vi "detect_spike_A_B_clean.vi"(6 "IO Module\\AI 1 Data N-3":i16, 9 "IO Module\\AI 1 Data N-2":i16, 10 "IO Module\\AI 1 Data N-1":i16, 11 "IO Module\\AI 1 Data N":i16) -> (3 "Numeric":i32, 5 "Read Ready A":bool, 7 "Read Ready B":bool)   [LabVIEW 2020]
panel:
  out "count_out":i16
  out "Read B 2":bool
  out "Read A 2":bool
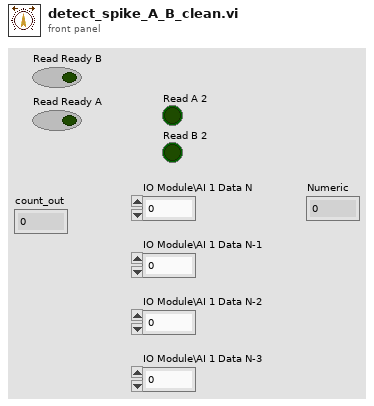
[diagram p1: front panel]
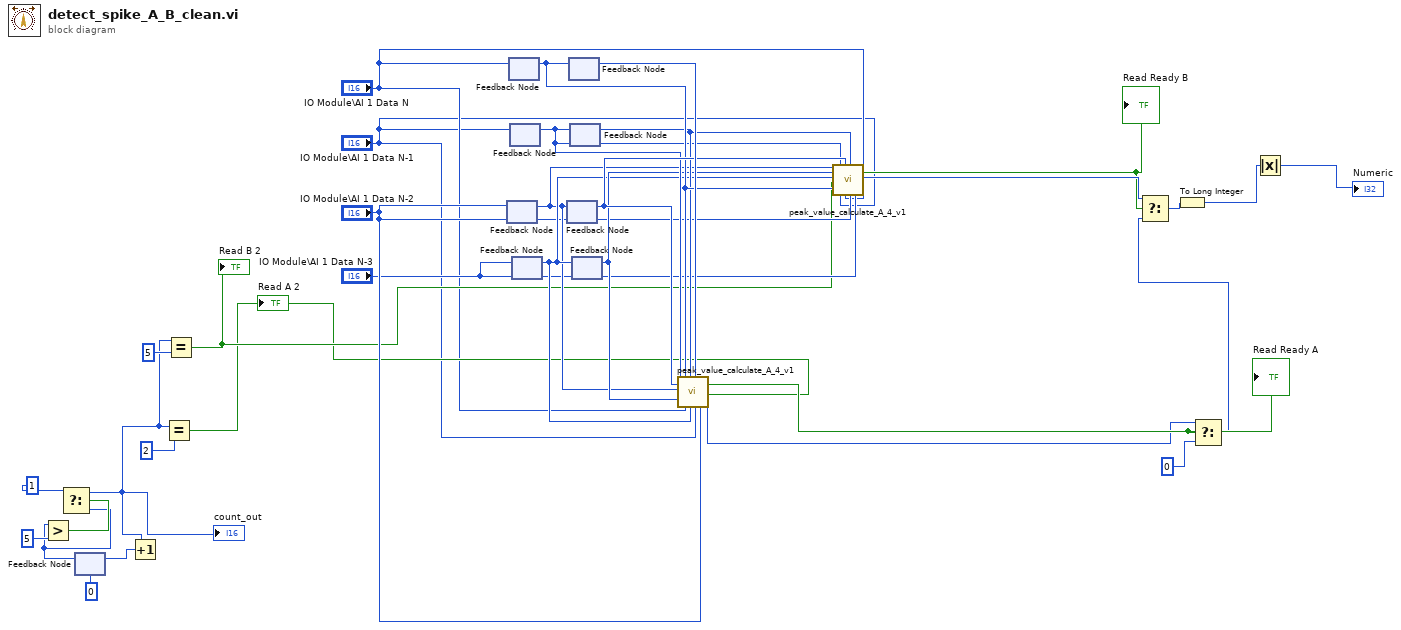
[diagram p0: block diagram]
diagram:
  n1 = feedback #1(i16 0) -> (w8:i16)
  n2 = Greater?(x=w8, y=i16 5 ("count")) -> (0:w12:bool)
  n3 = Select(t=i16 1, s=w12, f=w8) -> (s? t:f=w7:i16)
  "count_out" <- w7
  n4 = Increment(x=w7) -> (x+1=w10:i16)
  n5 = feedback-in #1(w10) -> ()
  n6 = Equal?(x=w7, y=i16 2) -> (x = y?=w16:bool)
  "Read A 2" <- w16
  n7 = Equal?(x=w7, y=i16 5) -> (x = y?=w17:bool)
  "Read B 2" <- w17
  n8 = feedback #2() -> (w22:i16)  [unwired: 1 in]
  n9 = feedback-in #2("IO Module\\AI 1 Data N-2") -> ()
  n10 = feedback #3() -> (w27:i16)  [unwired: 1 in]
  n11 = feedback-in #3("IO Module\\AI 1 Data N") -> ()
  n12 = feedback #4() -> (w25:i16)  [unwired: 1 in]
  n13 = feedback-in #4("IO Module\\AI 1 Data N-1") -> ()
  n14 = feedback #5() -> (w23:i16)  [unwired: 1 in]
  n15 = feedback-in #5("IO Module\\AI 1 Data N-3") -> ()
  n16 = feedback #6() -> (w28:i16)  [unwired: 1 in]
  n17 = feedback-in #6(w22) -> ()
  n18 = feedback #7() -> (w32:i16)  [unwired: 1 in]
  n19 = feedback-in #7(w27) -> ()
  n20 = feedback #8() -> (w26:i16)  [unwired: 1 in]
  n21 = feedback-in #8(w25) -> ()
  n22 = feedback #9() -> (w24:i16)  [unwired: 1 in]
  n23 = feedback-in #9(w23) -> ()
  n24 = call "peak_value_calculate_A_4_v1.vi"("IO Module\\AI 1 Data N-1 2"=w25, "IO Module\\AI 1 Data N-2 3"=w28, "IO Module\\AI 1 Data N-2 2"=w22, "Boolean in"=w16, "IO Module\\AI 1 Data N-3 2"=w24, "IO Module\\AI 1 Data N 3"=w27, "IO Module\\AI 1 Data N"="IO Module\\AI 1 Data N", "IO Module\\AI 1 Data N-1 3"=w26, "IO Module\\AI 1 Data N-3"=w23, "IO Module\\AI 1 Data N 2"=w32, "IO Module\\AI 1 Data N-1"="IO Module\\AI 1 Data N-1", "IO Module\\AI 1 Data N-2"="IO Module\\AI 1 Data N-2") -> ("Read Ready"=w29:bool, "Spike Value"=w4:i16)  [unwired: 6 in]
  "Read Ready A" <- w29
  n25 = call "peak_value_calculate_A_4_v1.vi"("IO Module\\AI 1 Data N-1 2"=w22, "IO Module\\AI 1 Data N-2 3"=w24, "IO Module\\AI 1 Data N-2 2"=w23, "Boolean in"=w17, "IO Module\\AI 1 Data N-3 2"=w27, "IO Module\\AI 1 Data N 3"=w25, "IO Module\\AI 1 Data N"="IO Module\\AI 1 Data N-1", "IO Module\\AI 1 Data N-1 3"=w28, "IO Module\\AI 1 Data N-3"="IO Module\\AI 1 Data N", "IO Module\\AI 1 Data N 2"=w26, "IO Module\\AI 1 Data N-1"="IO Module\\AI 1 Data N-2", "IO Module\\AI 1 Data N-2"="IO Module\\AI 1 Data N-3") -> ("Read Ready"=w14:bool, "Spike Value"=w15:i16)  [unwired: 6 in]
  "Read Ready B" <- w14
  n26 = Select(t=w4, s=w29, f=i16 0) -> (s? t:f=w6:i16)
  n27 = Select(t=w15, s=w14, f=w6) -> (s? t:f=w5:i16)
  n28 = To Long Integer(number=w5) -> (32bit integer=w30:i32)
  n29 = Absolute Value(x=w30) -> (abs(x)=→"Numeric":i32)
